vi "Default Behavior.vi"(0 "Start Stop Reactor Array":refnum<vi>, 1 "System Idle Array":refnum<vi>, 2 "Default Purge":refnum<vi>, 3 "Current Valve State":refnum<vi>, 4 "Current Locks":refnum<vi>, 5 "Reactor Name":string, 6 "Number of Reactors":i32, 7 "Stop Program":refnum<vi>, 8 "Valves Per Reactor":i32=6, 9 "Debug Mode":refnum<vi>, 10 "Lock Reentrance Rate":i32, 11 "Queue System":refnum<vi>, 12 "Pump Valves":i32[](array[numeric]), 13 "Queue JSON Object":refnum<vi>, 14 "Number of Shared Lines":i32, 16 "Reactor Selector":T1(ring)) -> ()   [LabVIEW 2021]
uses:
  7d1c9536-3f04-4bc7-9a02-fdf56edec875.vi
  a07f947c-fa61-40cd-9d4d-f5b80dcd4677.vi
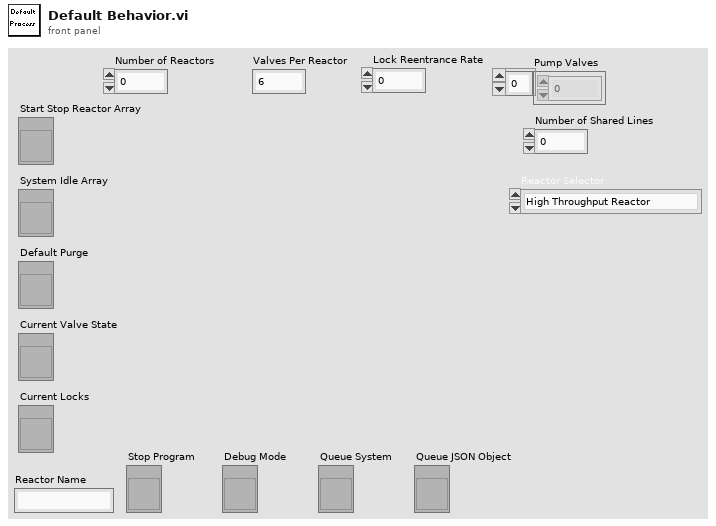
[diagram p1: front panel]
types:
  T1 = enum16{"High Throughput Reactor", "In Situ Reactor", "MLD Reactor"}
  T2 = enum16{"Lock", "Release", "Check", "Check All", "Release All"}
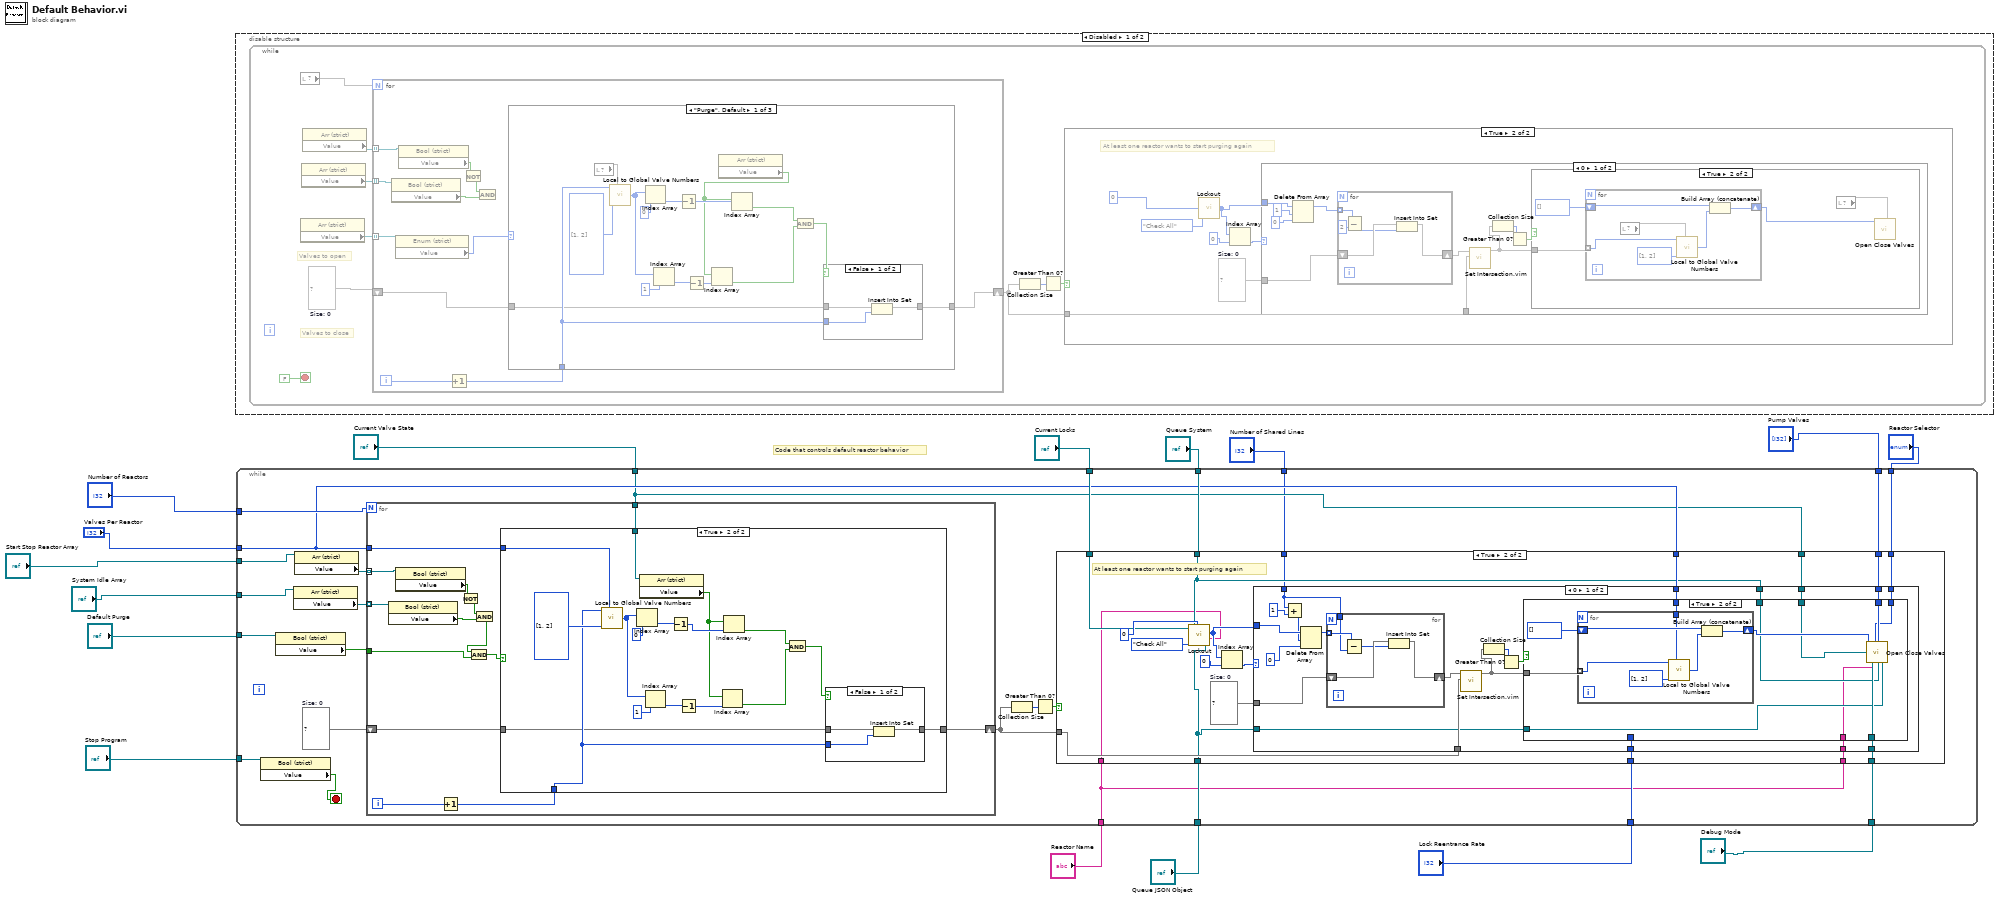
[diagram p0: block diagram]
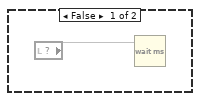
[diagram p2: hidden frame]
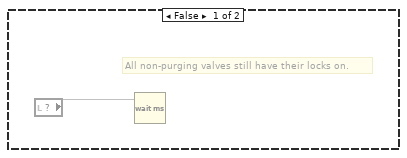
[diagram p3: hidden frame]
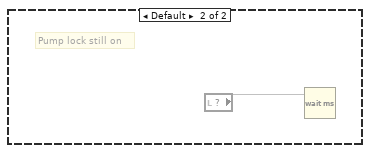
[diagram p4: hidden frame]
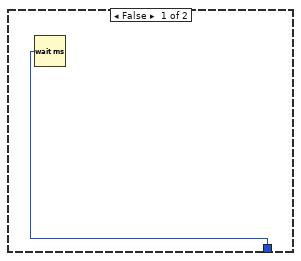
[diagram p9: hidden frame]
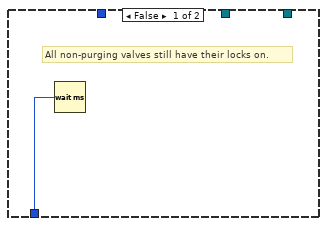
[diagram p10: hidden frame]
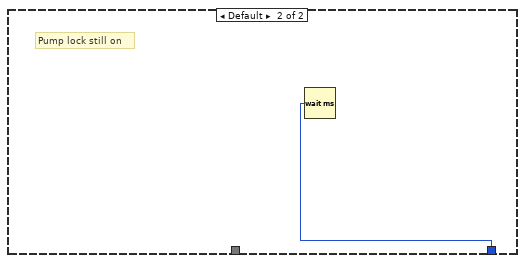
[diagram p11: hidden frame]
diagram:
  # "Code that controls default reactor behavior"
  n1 = disable-structure shown="Disabled" {
    frame Disabled {
      n2 = while {
        stop <- FALSE stop-if-true
        w22 = set{i32} {}  # Size: 0
        # "Valves to close"
        # "Valves to open"
        n3 = local read item#-1() -> (w25)
        n4 = property class="Arr (strict)"() -> (reference=w18:refnum<vi>, "Value"=w17:refnum<vi>[])  [unwired: 1 in, 2 out]
        n5 = property class="Arr (strict)"() -> ("Value"=w23:refnum<vi>[])  [unwired: 2 in, 2 out]
        n6 = property class="Arr (strict)"() -> ("Value"=w24:refnum<vi>[])  [unwired: 2 in, 2 out]
        n7 = for {
          N: w25 -> [_]
          tunnel: w24 -> [w77] mode=indexing
          tunnel: w23 -> [w76] mode=indexing
          shift-right: [w71] -> w19
          shift-left: w22 -> [w72]
          tunnel: w17 -> [w70] mode=indexing
          i -> [w79]
          n8 = property class="Bool (strict)"(reference=w76) -> ("Value"=w74:bool)  [unwired: 1 in, 2 out]
          n9 = property class="Enum (strict)"(reference=w70) -> ("Value"=w69:enum16{"Purge", "Pump", "Block"})  [unwired: 1 in, 2 out]
          n10 = property class="Bool (strict)"(reference=w77) -> ("Value"=w75:bool)  [unwired: 1 in, 2 out]
          n11 = Increment(x=w79) -> (x+1=w78:i32)
          n12 = Not(x=w75) -> (.not. x?=w73:bool)
          n13 = And(x=w73, y=w74) -> ()  [unwired: 1 out]
          n14 = case shown="\"Purge\", Default" w69 {
            tunnel: w78 -> [w90 _ _]
            tunnel: w72 -> [w81 w100 _]
            tunnel: [w80 w100 _] -> w71
            frame "Purge", Default {
              n15 = local read item#-1() -> (w95)
              n16 = call "Local to Global Valve Numbers.vi"("Reactor ID #"=w90, "List of Local Valves"=i32[] [1, 2], "Valves Per Reactor"=w95) -> ("List of Global Valves"=w85:i32[])  [unwired: 2 in]
              n17 = Index Array(array=w85, index=0) -> (element=w94:i32)
              n18 = Index Array(array=w85, index=1) -> (element=w87:i32)
              n19 = Decrement(x=w94) -> (x-1=w93:i32)
              n20 = Decrement(x=w87) -> (x-1=w88:i32)
              n21 = property class="Arr (strict)"() -> ("Value"=w86:bool[])  [unwired: 2 in, 2 out]
              n22 = Index Array(array=w86, index=w88) -> (element=w83:bool)
              n23 = Index Array(array=w86, index=w93) -> (element=w82:bool)
              n24 = And(x=w82, y=w83) -> (x .and. y?=w84:bool)
              n25 = case shown="False" w84 {
                tunnel: w90 -> [w97 _]
                tunnel: w81 -> [w98 w99]
                tunnel: [w96 w99] -> w80
                frame False {
                  n26 = Insert Into Set(10:w97, 11:w98) -> (3:w96:set{i32})  [unwired: 1 out]
                }
                frame True {
                  # "Purge on, do nothing"
                }
              }
            }
            frame "Pump" {
            }
            frame "Block" {
            }
          }
        }
        n27 = Collection Size(1:w19) -> (0:w20:i32)
        n28 = Greater Than 0?(x=w20) -> (x > 0?=w21:bool)
        n29 = case shown="True" w21 {
          tunnel: w19 -> [_ w34]
          frame False {
            n30 = local read item#-1() -> (w27)
            n31 = Wait (ms)(milliseconds to wait=w27) -> ()  [unwired: 1 out]
          }
          frame True {
            w35 = set{i32} {}  # Size: 0
            # "At least one reactor wants to start purging again"
            n32 = call "Lockout.vi"("ID"=0, "Request Type"=T2."Check All") -> ("Locks"=w32:refnum<vi>, "Queue System"=w30:refnum<vi>, "Locks Held"=w28:i32[], "JSON Queue"=w29:refnum<vi>)  [unwired: 1 in, 1 out]
            n33 = Index Array(array=w28, index=0) -> (element=w36:i32)
            n34 = case shown="0" w36 {
              tunnel: w28 -> [w47 _]
              tunnel: w35 -> [w43 _]
              tunnel: w34 -> [w41 _]
              frame 0 {
                n35 = Delete From Array(array=w47, length=1, index=0) -> (array with subset deleted=w44:i32[])  [unwired: 1 out]
                n36 = for {
                  tunnel: w44 -> [w64] mode=indexing
                  shift-right: [w66] -> w42
                  shift-left: w43 -> [w67]
                  n37 = Subtract(x=w64, y=2) -> (x-y=w65:i32)
                  n38 = Insert Into Set(10:w65, 11:w67) -> (3:w66:set{i32})  [unwired: 1 out]
                }
                n39 = call "Set Intersection.vim"("set 2"=w41, "set 1"=w42) -> ("intersection"=w40:set{i32})  [unwired: 9 in]
                n40 = Collection Size(1:w40) -> (0:w39:i32)
                n41 = Greater Than 0?(x=w39) -> (x > 0?=w38:bool)
                n42 = case shown="True" w38 {
                  tunnel: w40 -> [_ w56]
                  frame False {
                    # "All non-purging valves still have their locks on."
                    n43 = local read item#-1() -> (w48)
                    n44 = Wait (ms)(milliseconds to wait=w48) -> ()  [unwired: 1 out]
                  }
                  frame True {
                    n45 = for {
                      tunnel: w56 -> [w59] mode=indexing
                      shift-right: [w58] -> w51
                      shift-left: i32[] [] -> [w62]
                      n46 = local read item#-1() -> (w61)
                      n47 = call "Local to Global Valve Numbers.vi"("Reactor ID #"=w59, "List of Local Valves"=i32[] [1, 2], "Valves Per Reactor"=w61) -> ("List of Global Valves"=w57:i32[])  [unwired: 2 in]
                      n48 = Build Array (concatenate)(w62, w57) -> (w58:i32[])
                    }
                    n49 = local read item#-1() -> (w53)
                    n50 = call "Open Close Valves.vi"("Valves to Open"=w51, "Pump Valves"=w53) -> ("Current Valve State"=w52:refnum<vi>, "Debug Mode"=w49:refnum<vi>, "System Queue"=w54:refnum<vi>, "JSON Queue"=w50:refnum<vi>)  [unwired: 14 in]
                  }
                }
              }
              frame Default {
                # "Pump lock still on"
                n51 = local read item#-1() -> (w68)
                n52 = Wait (ms)(milliseconds to wait=w68) -> ()  [unwired: 1 out]
              }
            }
          }
        }
      }
    }
    frame Enabled {
    }
  }
  n53 = while {
    tunnel: "Number of Reactors" -> [w118]
    tunnel: "Start Stop Reactor Array" -> [w117]
    tunnel: "System Idle Array" -> [w116]
    tunnel: "Default Purge" -> [w114]
    tunnel: "Stop Program" -> [w112]
    tunnel: "Valves Per Reactor" -> [w108]
    tunnel: "Current Valve State" -> [w105]
    tunnel: "Current Locks" -> [w111]
    tunnel: "Queue System" -> [w110]
    tunnel: "Queue JSON Object" -> [w109]
    tunnel: "Lock Reentrance Rate" -> [w107]
    tunnel: "Debug Mode" -> [w106]
    tunnel: "Pump Valves" -> [w104]
    tunnel: "Number of Shared Lines" -> [w103]
    tunnel: "Reactor Name" -> [w102]
    tunnel: "Reactor Selector" -> [w101]
    stop <- w113 stop-if-true
    w122 = set{i32} {}  # Size: 0
    n54 = property class="Bool (strict)"(reference=w112) -> ("Value"=w113:bool)  [unwired: 1 in, 2 out]
    n55 = property class="Bool (strict)"(reference=w114) -> ("Value"=w115:bool)  [unwired: 1 in, 2 out]
    n56 = property class="Arr (strict)"(reference=w116) -> ("Value"=w123:refnum<vi>[])  [unwired: 1 in, 2 out]
    n57 = property class="Arr (strict)"(reference=w117) -> ("Value"=w124:refnum<vi>[])  [unwired: 1 in, 2 out]
    n58 = for {
      N: w118 -> [_]
      tunnel: w124 -> [w201] mode=indexing
      tunnel: w123 -> [w200] mode=indexing
      shift-right: [w193] -> w119
      shift-left: w122 -> [w194]
      tunnel: w115 -> [w192]
      tunnel: w108 -> [w191]
      tunnel: w105 -> [w190]
      i -> [w203]
      n59 = property class="Bool (strict)"(reference=w200) -> ("Value"=w198:bool)  [unwired: 1 in, 2 out]
      n60 = property class="Bool (strict)"(reference=w201) -> ("Value"=w199:bool)  [unwired: 1 in, 2 out]
      n61 = Increment(x=w203) -> (x+1=w202:i32)
      n62 = Not(x=w199) -> (.not. x?=w197:bool)
      n63 = And(x=w197, y=w198) -> (x .and. y?=w196:bool)
      n64 = And(x=w196, y=w192) -> (x .and. y?=w195:bool)
      n65 = case shown="True" w195 {
        tunnel: w202 -> [_ w217]
        tunnel: w194 -> [w204 w208]
        tunnel: [w204 w207] -> w193
        tunnel: w191 -> [_ w206]
        tunnel: w190 -> [_ w205]
        frame False {
        }
        frame True {
          n66 = call "Local to Global Valve Numbers.vi"("Reactor ID #"=w217, "List of Local Valves"=i32[] [1, 2], "Valves Per Reactor"=w206) -> ("List of Global Valves"=w212:i32[])  [unwired: 2 in]
          n67 = Index Array(array=w212, index=0) -> (element=w221:i32)
          n68 = property class="Arr (strict)"(reference=w205) -> ("Value"=w213:bool[])  [unwired: 1 in, 2 out]
          n69 = Index Array(array=w212, index=1) -> (element=w214:i32)
          n70 = Decrement(x=w221) -> (x-1=w220:i32)
          n71 = Decrement(x=w214) -> (x-1=w215:i32)
          n72 = Index Array(array=w213, index=w215) -> (element=w210:bool)
          n73 = Index Array(array=w213, index=w220) -> (element=w209:bool)
          n74 = And(x=w209, y=w210) -> (x .and. y?=w211:bool)
          n75 = case shown="False" w211 {
            tunnel: w217 -> [w223 _]
            tunnel: w208 -> [w224 w225]
            tunnel: [w222 w225] -> w207
            frame False {
              n76 = Insert Into Set(10:w223, 11:w224) -> (3:w222:set{i32})  [unwired: 1 out]
            }
            frame True {
              # "Purge on, do nothing"
            }
          }
        }
      }
    }
    n77 = Collection Size(1:w119) -> (0:w120:i32)
    n78 = Greater Than 0?(x=w120) -> (x > 0?=w121:bool)
    n79 = case shown="True" w121 {
      tunnel: w119 -> [_ w141]
      tunnel: w111 -> [_ w137]
      tunnel: w110 -> [_ w132]
      tunnel: w109 -> [_ w131]
      tunnel: w108 -> [_ w136]
      tunnel: w107 -> [w125 w135]
      tunnel: w106 -> [_ w134]
      tunnel: w105 -> [_ w133]
      tunnel: w104 -> [_ w130]
      tunnel: w103 -> [_ w129]
      tunnel: w102 -> [_ w128]
      tunnel: w102 -> [_ w127]
      tunnel: w101 -> [_ w126]
      frame False {
        n80 = Wait (ms)(milliseconds to wait=w125) -> ()  [unwired: 1 out]
      }
      frame True {
        w142 = set{i32} {}  # Size: 0
        # "At least one reactor wants to start purging again"
        n81 = call "Lockout.vi"("Locks"=w137, "ID"=0, "Queue System"=w132, "Request Type"=T2."Check All", "Reactor Name"=w128, "JSON Queue"=w131) -> ("Locks Held"=w138:i32[])  [unwired: 1 in, 1 out]
        n82 = Index Array(array=w138, index=0) -> (element=w143:i32)
        n83 = case shown="0" w143 {
          tunnel: w138 -> [w165 _]
          tunnel: w142 -> [w162 _]
          tunnel: w141 -> [w160 _]
          tunnel: w136 -> [w156 _]
          tunnel: w135 -> [w155 w189]
          tunnel: w134 -> [w154 _]
          tunnel: w133 -> [w153 _]
          tunnel: w132 -> [w152 _]
          tunnel: w131 -> [w151 _]
          tunnel: w130 -> [w150 _]
          tunnel: w129 -> [w147 _]
          tunnel: w127 -> [w146 _]
          tunnel: w126 -> [w145 _]
          frame 0 {
            n84 = Add(x=w147, y=1 ("length")) -> (x+y=w148:i32)
            n85 = Delete From Array(array=w165, length=w148, index=0) -> (array with subset deleted=w163:i32[])  [unwired: 1 out]
            n86 = for {
              tunnel: w163 -> [w185] mode=indexing
              shift-right: [w187] -> w161
              shift-left: w162 -> [w188]
              tunnel: w147 -> [w184]
              n87 = Subtract(x=w185, y=w184) -> (x-y=w186:i32)
              n88 = Insert Into Set(10:w186, 11:w188) -> (3:w187:set{i32})  [unwired: 1 out]
            }
            n89 = call "Set Intersection.vim"("set 2"=w160, "set 1"=w161) -> ("intersection"=w159:set{i32})  [unwired: 9 in]
            n90 = Collection Size(1:w159) -> (0:w158:i32)
            n91 = Greater Than 0?(x=w158) -> (x > 0?=w157:bool)
            n92 = case shown="True" w157 {
              tunnel: w159 -> [_ w177]
              tunnel: w156 -> [_ w174]
              tunnel: w155 -> [w166 _]
              tunnel: w154 -> [_ w173]
              tunnel: w153 -> [_ w172]
              tunnel: w152 -> [_ w171]
              tunnel: w151 -> [_ w170]
              tunnel: w150 -> [_ w169]
              tunnel: w146 -> [_ w168]
              tunnel: w145 -> [_ w167]
              frame False {
                # "All non-purging valves still have their locks on."
                n93 = Wait (ms)(milliseconds to wait=w166) -> ()  [unwired: 1 out]
              }
              frame True {
                n94 = for {
                  tunnel: w177 -> [w181] mode=indexing
                  shift-right: [w180] -> w175
                  shift-left: i32[] [] -> [w183]
                  tunnel: w174 -> [w178]
                  n95 = call "Local to Global Valve Numbers.vi"("Reactor ID #"=w181, "List of Local Valves"=i32[] [1, 2], "Valves Per Reactor"=w178) -> ("List of Global Valves"=w179:i32[])  [unwired: 2 in]
                  n96 = Build Array (concatenate)(w183, w179) -> (w180:i32[])
                }
                n97 = call "Open Close Valves.vi"("Valves to Open"=w175, "Current Valve State"=w172, "Debug Mode"=w173, "Reactor Name"=w168, "Reactor Selector"=w167, "Pump Valves"=w169, "System Queue"=w171, "JSON Queue"=w170) -> ()  [unwired: 12 in]
              }
            }
          }
          frame Default {
            # "Pump lock still on"
            n98 = Wait (ms)(milliseconds to wait=w189) -> ()  [unwired: 1 out]
          }
        }
      }
    }
  }
